vi "Begin.vi"(8 "error in":errorcluster) -> (0 "error out":errorcluster)   [LabVIEW 2019]
doc: "Called before other user functions, this VI is expected to open initial I/O refnums, load in file data, and do all program initialization. Notice that the <B>error out</B> terminal is simply used for data flow. Wiring it to other structures or subVIs ensures that this VI runs first."
uses:
  <vilib>/Rock Robotics/WPI/DriverStation/WPI_DriverStationRobotMode2.ctl
  <vilib>/Rock Robotics/WPI/Joystick/WPI_JoystickDeviceEnum.ctl
  <vilib>/Rock Robotics/SystemInterfaces/DIO/FPGA_DIOPWMChannel.ctl
  <vilib>/Rock Robotics/SystemInterfaces/DIO/FPGA_DIORelayChannel.ctl
  <vilib>/Rock Robotics/WPI/Solenoid/WPI_SolenoidChannel.ctl
  <vilib>/Rock Robotics/SystemInterfaces/DIO/FPGA_DIOChannel.ctl
  <vilib>/Rock Robotics/SystemInterfaces/i2clib/i2c_bus.ctl
  <vilib>/Rock Robotics/SystemInterfaces/AI/FPGA_AIChannel.ctl
  <vilib>/Rock Robotics/SystemInterfaces/spilib/spi_bus.ctl
  Robot Global Data.vi
  <vilib>/Rock Robotics/WPI/MotorControl/WPI_MotorControlOpen SPARK.vi
  <vilib>/Rock Robotics/WPI/MotorControl/WPI_MotorControlOpen VictorSPX.vi
  <vilib>/Rock Robotics/WPI/Solenoid/WPI_SolenoidOpenSingle.vi
  <vilib>/Rock Robotics/WPI/Counter/WPI_CounterDigitalInputToDigitalSource.vi
  Program Files/navX.Library.v2/navX Library v2/IO/Open/Z900_navX_Open_SPI.vi
  Program Files/navX.Library.v2/navX Library v2/navX Library v2.lvlib
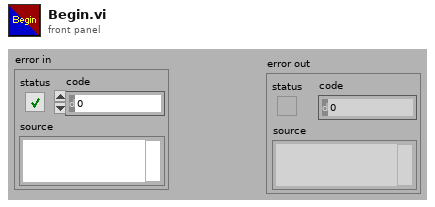
[diagram p1: front panel]
types:
  T1 = typedef "WPI_DriverStationRobotMode2.ctl" = enum16{"Autonomous Disabled", "Autonomous Enabled", "Teleop Disabled", "Teleop Enabled", "Disconnected", "Finish", "Test Disabled", "Test Enabled", "Emergency Stopped"}
  T2 = typedef "WPI_JoystickDeviceEnum.ctl" = enum16{"USB 0", "USB 1", "USB 2", "USB 3", "USB 4", "USB 5"}
  T3 = typedef "FPGA_DIORelayChannel.ctl" = enum8{"Relay 0", "Relay 1", "Relay 2", "Relay 3", "Invalid"}
  T4 = typedef "WPI_SolenoidChannel.ctl" = enum8{"Solenoid 0", "Solenoid 1", "Solenoid 2", "Solenoid 3", "Solenoid 4", "Solenoid 5", "Solenoid 6", "Solenoid 7", "Invalid"}
  T5 = typedef "FPGA_DIOPWMChannel.ctl" = enum8{"PWM 0", "PWM 1", "PWM 2", "PWM 3", "PWM 4", "PWM 5", "PWM 6", "PWM 7", "PWM 8", "PWM 9", "PWM MXP 0", "PWM MXP 1", "PWM MXP 2", "PWM MXP 3", "PWM MXP 4", "PWM MXP 5", "PWM MXP 6", "PWM MXP 7", "PWM MXP 8", "PWM MXP 9", "Invalid"}
  T6 = typedef "FPGA_AIChannel.ctl" = enum8{"AI 0", "AI 1", "AI 2", "AI 3", "AI MXP 0", "AI MXP 1", "AI MXP 2", "AI MXP 3", "Invalid"}
  T7 = typedef "spi_bus.ctl" = enum16{"SPI On-Board, CS0", "SPI On-Board, CS1", "SPI On-Board, CS2", "SPI On-Board, CS3", "SPI MXP", "Invalid"}
  T8 = typedef "i2c_bus.ctl" = enum16{"I2C On-Board", "I2C MXP", "Invalid"}
  T9 = typedef "WPI_JoystickDevRef.ctl" = cluster{"Device":T2}
  T10 = typedef "WPI_MotorControlDeviceRef.ctl" = cluster{"DeviceStatus":errorcluster, "Type":T11, "PWM":cluster{"PWM Channel":T5, "DeadBand":T12}, "CAN":cluster{"Device Number":u8, "SetOutput VI Ref":variant, "GetOutput VI Ref":variant, "Enable VI Ref":variant, "Disable VI Ref":variant, "Data":variant}, "Invert":bool, "DIO PWM":cluster{"PWM \"Enable\" Channel":T5, "DIOChannel":T13, "PWM Rate":dbl}}
  T11 = typedef "WPI_MotorControlType.ctl" = enum16{"PWM", "CAN", "DIO PWM"}
  T12 = typedef "WPI_PWMDeadband.ctl" = cluster{"Name":string, "maxPositivePwm":i32, "minPositivePwm":i32, "centerPwm":i32, "maxNegativePwm":i32, "minNegativePwm":i32, "angularRange":u16}
  T13 = typedef "FPGA_DIOChannel.ctl" = enum8{"DIO 0", "DIO 1", "DIO 2", "DIO 3", "DIO 4", "DIO 5", "DIO 6", "DIO 7", "DIO 8", "DIO 9", "DIO MXP 0", "DIO MXP 1", "DIO MXP 2", "DIO MXP 3", "DIO MXP 4", "DIO MXP 5", "DIO MXP 6", "DIO MXP 7", "DIO MXP 8", "DIO MXP 9", "DIO MXP 10", "DIO MXP 11", "DIO MXP 12", "DIO MXP 13", "DIO MXP 14", "DIO MXP 15", "SPI Port CS1", "SPI Port CS2", "SPI Port CS3", "SPI Port MISO", "SPI Port MOSI", "Invalid"}
  T14 = typedef "WPI_RelayDevRef.ctl" = cluster{"DevStatus":errorcluster, "Relay Channel":T3, "Relay Direction":T15}
  T15 = typedef "WPI_RelayDirection.ctl" = enum16{"Both directions", "Forward only", "Reverse only"}
  T16 = typedef "WPI_CompressorDevRef.ctl" = cluster{"DevStatus":errorcluster, "Pneumatics Control Module":u8}
  T17 = typedef "WPI_SolenoidDevRef.ctl" = cluster{"DevStatus":errorcluster, "Pneumatics Control Module":u8, "Forward Solenoid Channel":T4, "Reverse Solenoid Channel":T4}
  T18 = typedef "WPI_AnalogChannelDevRef.ctl" = cluster{"DevStatus":errorcluster, "Analog Channel":T6}
  T19 = typedef "WPI_DigitalInputDevRef.ctl" = cluster{"DevStatus":errorcluster, "DIO Channel":T13}
  T20 = typedef "Color Sensor V3 DevRef.ctl" = cluster{"I2CDevRef":T21}
  T21 = typedef "WPI_I2CDevRef.ctl" = cluster{"DevStatus":errorcluster, "Device Address":u8, "Handle":i32, "I2C Bus":T8}
  T22 = typedef "FPGA_CounterEncoderSourceConvertionLVSourceType.ctl" = cluster{"DevStatus":errorcluster, "AnalogTriggerMode?":bool, "DigitalMode":cluster{"DIO Channel":T23}, "AnalogTriggerMode":cluster{"AnalogTriggerIndex":T24, "OutputType":T25}}
  T23 = typedef "FPGA_DIODigitalSourceChannel.ctl" = enum8{"DIO 0", "DIO 1", "DIO 2", "DIO 3", "DIO 4", "DIO 5", "DIO 6", "DIO 7", "DIO 8", "DIO 9", "DIO MXP 0", "DIO MXP 1", "DIO MXP 2", "DIO MXP 3", "DIO MXP 4", "DIO MXP 5", "DIO MXP 6", "DIO MXP 7", "DIO MXP 8", "DIO MXP 9", "DIO MXP 10", "DIO MXP 11", "DIO MXP 12", "DIO MXP 13", "DIO MXP 14", "DIO MXP 15", "SPI Port CS1", "SPI Port CS2", "SPI Port CS3", "SPI Port MISO", "SPI Port MOSI", "Disabled"}
  T24 = typedef "FPGA_AnalogTriggerIndex.ctl" = enum8{"Trig 0", "Trig 1", "Trig 2", "Trig 3", "Trig 4", "Trig 5", "Trig 6", "Trig 7", "Invalid"}
  T25 = typedef "FPGA_AnalogTriggerOutType.ctl" = enum16{"InWindow", "TriggerState", "Rising", "Falling"}
  T26 = typedef "WPI_EncoderDevRef.ctl" = cluster{"DevStatus":errorcluster, "EncoderIndex":T27, "CounterIndex":T28, "DistancePerCount":dbl, "Decoding Type":T29}
  T27 = typedef "FPGA_EncoderIdx.ctl" = enum8{"Enc 0", "Enc 1", "Enc 2", "Enc 3", "Enc 4", "Enc 5", "Enc 6", "Enc 7", "Invalid"}
  T28 = typedef "FPGA_CounterCtrSystemIndex.ctl" = enum8{"Ctr 0", "Ctr 1", "Ctr 2", "Ctr 3", "Ctr 4", "Ctr 5", "Ctr 6", "Ctr 7", "Invalid"}
  T29 = typedef "WPI_EncoderType.ctl" = enum16{"1x", "2x", "4x"}
  T30 = typedef "navX Library v2.lvlib/Z900_navX_DeviceTypeDef.ctl" = cluster{"Interface":cluster{"Protocol":T31, "Update Rate (4Hz-100Hz)":u8, "navX Open TypeDef":variant}, "Notify Packet":refnum<notifier>, "Loop VI Refnum":refnum<vi>, "Ready to Close Occurrence Refnum":refnum<k4>}
  T31 = typedef "navX Library v2.lvlib/Z900_navX_ProtocolTypeDef.ctl" = enum16{"SERIAL", "I2C", "SPI"}
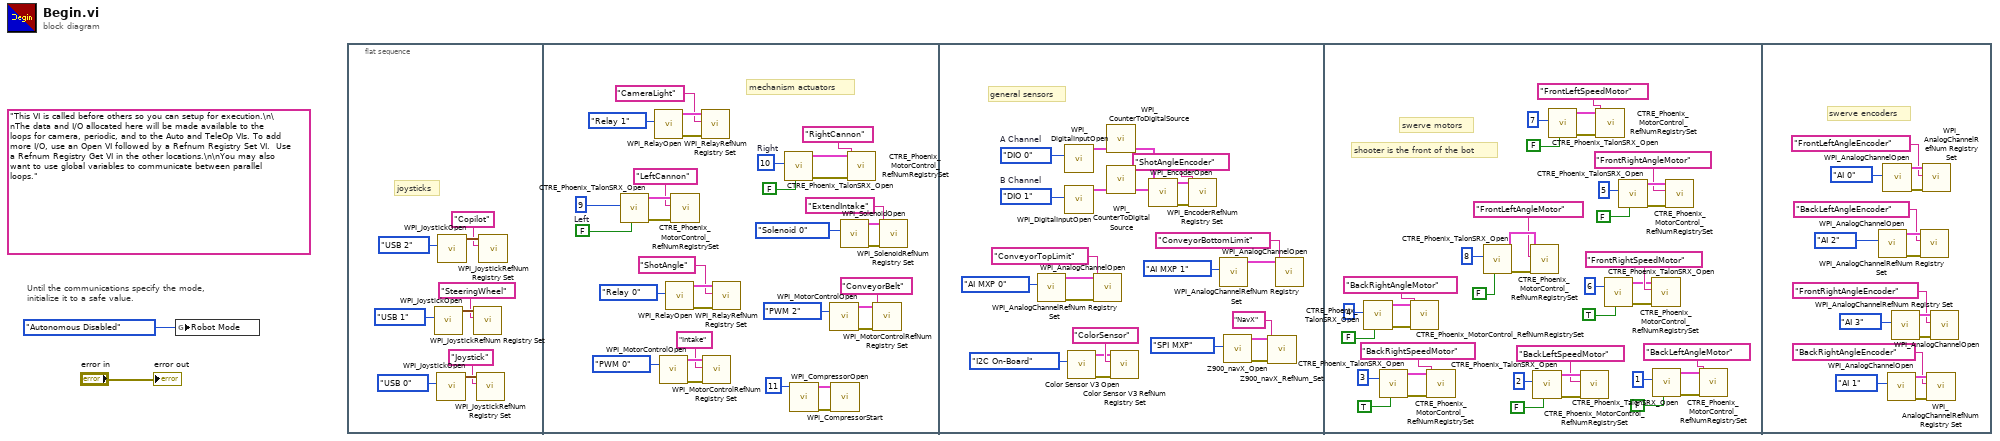
[diagram p0: block diagram]
diagram:
  (unwired) "This VI is called before others so you can setup for execution.\n\nThe data and I/O allocated here will be made available to the loops for camera, periodic, and to the Auto and TeleOp VIs. To add more I/O, use an Open VI followed by a Refnum Registry Set VI.  Use a Refnum Registry Get VI in the other locations.\n\nYou may also want to use global variables to communicate between parallel loops."
  # "Until the communications specify the mode,\ninitialize it to a safe value."
  n1 = global write "Robot Global Data.vi" "Robot Mode"(WPI_DriverStationRobotMode2."Autonomous Disabled" ("Robot Mode")) -> ()
  n2 = flat-sequence {
    frame #0 {
      # "joysticks"
      n3 = call <vilib>:"WPI_JoystickOpen.vi"("JoystickDevice"=WPI_JoystickDeviceEnum."USB 1") -> ("JoystickDevRef"=w7:T9)  [unwired: 10 in]
      n4 = call <vilib>:"WPI_JoystickOpen.vi"("JoystickDevice"=WPI_JoystickDeviceEnum."USB 0") -> ("JoystickDevRef"=w8:T9)  [unwired: 10 in]
      n5 = call <vilib>:"WPI_JoystickOpen.vi"("JoystickDevice"=WPI_JoystickDeviceEnum."USB 2") -> ("JoystickDevRef"=w11:T9)  [unwired: 10 in]
      n6 = call <vilib>:"WPI_JoystickRefNum Registry Set.vi"("refnum name"="SteeringWheel", "JoystickDevRef"=w7) -> ()  [unwired: 8 in, 2 out]
      n7 = call <vilib>:"WPI_JoystickRefNum Registry Set.vi"("refnum name"="Joystick", "JoystickDevRef"=w8) -> ()  [unwired: 8 in, 2 out]
      n8 = call <vilib>:"WPI_JoystickRefNum Registry Set.vi"("refnum name"="Copilot", "JoystickDevRef"=w11) -> ()  [unwired: 8 in, 2 out]
    }
    frame #1 {
      w43 = u8 9  # Left
      w44 = u8 10  # Right
      # "mechanism actuators"
      n9 = call <vilib>:"CTRE_Phoenix_TalonSRX_Open.vi"("Invert"=FALSE, "Device Number"=w43) -> ("error out"=w39:errorcluster, "CAN Talon SRX Ref"=w40:T10)  [unwired: 8 in]
      n10 = call <vilib>:"WPI_RelayOpen.vi"("Relay Channel"=FPGA_DIORelayChannel."Relay 1") -> ("error out"=w18:errorcluster, "RelayDevRef"=w17:T14)  [unwired: 9 in]
      n11 = call-poly <vilib>:"WPI_MotorControlOpen.vi"("PWM Channel"=FPGA_DIOPWMChannel."PWM 0") -> ("error out"=w34:errorcluster, "MotorControlDeviceRef"=w33:T10)  [unwired: 9 in]
      n12 = call <vilib>:"WPI_RelayOpen.vi"("Relay Channel"=FPGA_DIORelayChannel."Relay 0") -> ("error out"=w26:errorcluster, "RelayDevRef"=w25:T14)  [unwired: 9 in]
      n13 = call <vilib>:"CTRE_Phoenix_MotorControl_RefNumRegistrySet.vi"("error in (no error)"=w39, "refnum name"="LeftCannon", "PhoenixMotorControlDevRef"=w40) -> ()  [unwired: 7 in, 2 out]
      n14 = call <vilib>:"WPI_RelayRefNum Registry Set.vi"("error in (no error)"=w18, "refnum name"="CameraLight", "RelayDevRef"=w17) -> ()  [unwired: 7 in, 2 out]
      n15 = call <vilib>:"WPI_MotorControlRefNum Registry Set.vi"("error in (no error)"=w34, "refnum name"="Intake", "MotorControlDevRef"=w33) -> ()  [unwired: 7 in, 2 out]
      n16 = call <vilib>:"WPI_RelayRefNum Registry Set.vi"("error in (no error)"=w26, "refnum name"="ShotAngle", "RelayDevRef"=w25) -> ()  [unwired: 7 in, 2 out]
      n17 = call <vilib>:"CTRE_Phoenix_TalonSRX_Open.vi"("Invert"=FALSE, "Device Number"=w44) -> ("error out"=w36:errorcluster, "CAN Talon SRX Ref"=w37:T10)  [unwired: 8 in]
      n18 = call <vilib>:"WPI_CompressorOpen.vi"("Pneumatics Control Module (0)"=u8 11) -> ("CompressorDevRef"=w13:T16, "error out"=w12:errorcluster)  [unwired: 13 in]
      n19 = call-poly <vilib>:"WPI_MotorControlOpen.vi"("PWM Channel"=FPGA_DIOPWMChannel."PWM 2") -> ("error out"=w30:errorcluster, "MotorControlDeviceRef"=w29:T10)  [unwired: 9 in]
      n20 = call <vilib>:"WPI_CompressorStart.vi"("error in (no error)"=w12, "CompressorDevRef"=w13) -> ()  [unwired: 8 in, 2 out]
      n21 = call-poly <vilib>:"WPI_SolenoidOpen.vi"("Solenoid Channel"=WPI_SolenoidChannel."Solenoid 0") -> ("error out"=w21:errorcluster, "SolenoidDevRef"=w22:T17)  [unwired: 9 in]
      n22 = call <vilib>:"CTRE_Phoenix_MotorControl_RefNumRegistrySet.vi"("error in (no error)"=w36, "refnum name"="RightCannon", "PhoenixMotorControlDevRef"=w37) -> ()  [unwired: 7 in, 2 out]
      n23 = call <vilib>:"WPI_MotorControlRefNum Registry Set.vi"("error in (no error)"=w30, "refnum name"="ConveyorBelt", "MotorControlDevRef"=w29) -> ()  [unwired: 7 in, 2 out]
      n24 = call <vilib>:"WPI_SolenoidRefNum Registry Set.vi"("error in (no error)"=w21, "refnum name"="ExtendIntake", "SolenoidDevRef"=w22) -> ()  [unwired: 7 in, 2 out]
    }
    frame #2 {
      w68 = FPGA_DIOChannel."DIO 1"  # B Channel
      w67 = FPGA_DIOChannel."DIO 0"  # A Channel
      # "general sensors"
      n25 = call <vilib>:"WPI_AnalogChannelOpen.vi"("Analog Channel"=FPGA_AIChannel."AI MXP 0") -> ("error out"=w54:errorcluster, "AIDeviceRef"=w53:T18)  [unwired: 9 in]
      n26 = call <vilib>:"WPI_DigitalInputOpen.vi"("DIO Channel"=w67) -> ("DigitalInputDevRef"=w64:T19)  [unwired: 1 in, 9 out]
      n27 = call <vilib>:"WPI_DigitalInputOpen.vi"("DIO Channel"=w68) -> ("DigitalInputDevRef"=w65:T19)  [unwired: 1 in, 9 out]
      n28 = call <vilib>:"Color Sensor V3 Open.vi"("I2C Bus"=i2c_bus."I2C On-Board") -> ("error out"=w58:errorcluster, "ColorSensorDevRef"=w57:T20)  [unwired: 9 in]
      n29 = call <vilib>:"WPI_AnalogChannelRefNum Registry Set.vi"("error in (no error)"=w54, "refnum name"="ConveyorTopLimit", "AIDeviceRef"=w53) -> ()  [unwired: 7 in, 2 out]
      n30 = call-poly <vilib>:"WPI_CounterToDigitalSource.vi"("DigitalInputDevRef"=w64) -> ("Digital Source"=w63:T22)  [unwired: 6 out]
      n31 = call-poly <vilib>:"WPI_CounterToDigitalSource.vi"("DigitalInputDevRef"=w65) -> ("Digital Source"=w66:T22)  [unwired: 6 out]
      n32 = call <vilib>:"Color Sensor V3 RefNum Registry Set.vi"("error in (no error)"=w58, "refnum name"="ColorSensor", "ColorSensorDevRef"=w57) -> ()  [unwired: 7 in, 2 out]
      n33 = call <vilib>:"WPI_EncoderOpen.vi"("BSource"=w66, "ASource"=w63) -> ("error out"=w62:errorcluster, "EncoderDevRef"=w61:T26)  [unwired: 6 in, 2 out]
      n34 = call <vilib>:"WPI_EncoderRefNum Registry Set.vi"("error in (no error)"=w62, "refnum name"="ShotAngleEncoder", "EncoderDevRef"=w61) -> ()  [unwired: 7 in, 2 out]
      n35 = call <vilib>:"WPI_AnalogChannelOpen.vi"("Analog Channel"=FPGA_AIChannel."AI MXP 1") -> ("AIDeviceRef"=w46:T18)  [unwired: 9 in, 1 out]
      n36 = call-poly "Z900_navX_Open.vi"("SPI Bus"=spi_bus."SPI MXP") -> ("error out"=w48:errorcluster, "navX Device"=w51:T30)  [unwired: 9 in]
      n37 = call "Z900_navX_RefNum_Set.vi"("error in (no error)"=w48, "refnum name"="NavX", "navX Device"=w51) -> ()  [unwired: 7 in, 2 out]
      n38 = call <vilib>:"WPI_AnalogChannelRefNum Registry Set.vi"("refnum name"="ConveyorBottomLimit", "AIDeviceRef"=w46) -> ()  [unwired: 8 in, 2 out]
    }
    frame #3 {
      # "shooter is the front of the bot"
      # "swerve motors"
      n39 = call <vilib>:"CTRE_Phoenix_TalonSRX_Open.vi"("Invert"=FALSE, "Device Number"=u8 4) -> ("error out"=w88:errorcluster, "CAN Talon SRX Ref"=w87:T10)  [unwired: 8 in]
      n40 = call <vilib>:"CTRE_Phoenix_TalonSRX_Open.vi"("Invert"=TRUE, "Device Number"=u8 3) -> ("error out"=w103:errorcluster, "CAN Talon SRX Ref"=w104:T10)  [unwired: 8 in]
      n41 = call <vilib>:"CTRE_Phoenix_MotorControl_RefNumRegistrySet.vi"("error in (no error)"=w88, "refnum name"="BackRightAngleMotor", "PhoenixMotorControlDevRef"=w87) -> ()  [unwired: 7 in, 2 out]
      n42 = call <vilib>:"CTRE_Phoenix_MotorControl_RefNumRegistrySet.vi"("error in (no error)"=w103, "refnum name"="BackRightSpeedMotor", "PhoenixMotorControlDevRef"=w104) -> ()  [unwired: 7 in, 2 out]
      n43 = call <vilib>:"CTRE_Phoenix_TalonSRX_Open.vi"("Invert"=FALSE, "Device Number"=u8 8) -> ("error out"=w76:errorcluster, "CAN Talon SRX Ref"=w75:T10)  [unwired: 8 in]
      n44 = call <vilib>:"CTRE_Phoenix_MotorControl_RefNumRegistrySet.vi"("error in (no error)"=w76, "refnum name"="FrontLeftAngleMotor", "PhoenixMotorControlDevRef"=w75) -> ()  [unwired: 7 in, 2 out]
      n45 = call <vilib>:"CTRE_Phoenix_TalonSRX_Open.vi"("Invert"=FALSE, "Device Number"=u8 2) -> ("error out"=w94:errorcluster, "CAN Talon SRX Ref"=w95:T10)  [unwired: 8 in]
      n46 = call <vilib>:"CTRE_Phoenix_TalonSRX_Open.vi"("Invert"=FALSE, "Device Number"=u8 7) -> ("error out"=w92:errorcluster, "CAN Talon SRX Ref"=w93:T10)  [unwired: 8 in]
      n47 = call <vilib>:"CTRE_Phoenix_MotorControl_RefNumRegistrySet.vi"("error in (no error)"=w94, "refnum name"="BackLeftSpeedMotor", "PhoenixMotorControlDevRef"=w95) -> ()  [unwired: 7 in, 2 out]
      n48 = call <vilib>:"CTRE_Phoenix_MotorControl_RefNumRegistrySet.vi"("error in (no error)"=w92, "refnum name"="FrontLeftSpeedMotor", "PhoenixMotorControlDevRef"=w93) -> ()  [unwired: 7 in, 2 out]
      n49 = call <vilib>:"CTRE_Phoenix_TalonSRX_Open.vi"("Invert"=TRUE, "Device Number"=u8 6) -> ("error out"=w101:errorcluster, "CAN Talon SRX Ref"=w102:T10)  [unwired: 8 in]
      n50 = call <vilib>:"CTRE_Phoenix_TalonSRX_Open.vi"("Invert"=FALSE, "Device Number"=u8 5) -> ("error out"=w86:errorcluster, "CAN Talon SRX Ref"=w85:T10)  [unwired: 8 in]
      n51 = call <vilib>:"CTRE_Phoenix_MotorControl_RefNumRegistrySet.vi"("error in (no error)"=w101, "refnum name"="FrontRightSpeedMotor", "PhoenixMotorControlDevRef"=w102) -> ()  [unwired: 7 in, 2 out]
      n52 = call <vilib>:"CTRE_Phoenix_TalonSRX_Open.vi"("Invert"=FALSE, "Device Number"=u8 1) -> ("error out"=w78:errorcluster, "CAN Talon SRX Ref"=w77:T10)  [unwired: 8 in]
      n53 = call <vilib>:"CTRE_Phoenix_MotorControl_RefNumRegistrySet.vi"("error in (no error)"=w86, "refnum name"="FrontRightAngleMotor", "PhoenixMotorControlDevRef"=w85) -> ()  [unwired: 7 in, 2 out]
      n54 = call <vilib>:"CTRE_Phoenix_MotorControl_RefNumRegistrySet.vi"("error in (no error)"=w78, "refnum name"="BackLeftAngleMotor", "PhoenixMotorControlDevRef"=w77) -> ()  [unwired: 7 in, 2 out]
    }
    frame #4 {
      # "swerve encoders"
      n55 = call <vilib>:"WPI_AnalogChannelOpen.vi"("Analog Channel"=FPGA_AIChannel."AI 2") -> ("error out"=w119:errorcluster, "AIDeviceRef"=w120:T18)  [unwired: 9 in]
      n56 = call <vilib>:"WPI_AnalogChannelOpen.vi"("Analog Channel"=FPGA_AIChannel."AI 0") -> ("error out"=w123:errorcluster, "AIDeviceRef"=w124:T18)  [unwired: 9 in]
      n57 = call <vilib>:"WPI_AnalogChannelOpen.vi"("Analog Channel"=FPGA_AIChannel."AI 1") -> ("error out"=w111:errorcluster, "AIDeviceRef"=w112:T18)  [unwired: 9 in]
      n58 = call <vilib>:"WPI_AnalogChannelOpen.vi"("Analog Channel"=FPGA_AIChannel."AI 3") -> ("error out"=w115:errorcluster, "AIDeviceRef"=w116:T18)  [unwired: 9 in]
      n59 = call <vilib>:"WPI_AnalogChannelRefNum Registry Set.vi"("error in (no error)"=w119, "refnum name"="BackLeftAngleEncoder", "AIDeviceRef"=w120) -> ()  [unwired: 7 in, 2 out]
      n60 = call <vilib>:"WPI_AnalogChannelRefNum Registry Set.vi"("error in (no error)"=w123, "refnum name"="FrontLeftAngleEncoder", "AIDeviceRef"=w124) -> ()  [unwired: 7 in, 2 out]
      n61 = call <vilib>:"WPI_AnalogChannelRefNum Registry Set.vi"("error in (no error)"=w111, "refnum name"="BackRightAngleEncoder", "AIDeviceRef"=w112) -> ()  [unwired: 7 in, 2 out]
      n62 = call <vilib>:"WPI_AnalogChannelRefNum Registry Set.vi"("error in (no error)"=w115, "refnum name"="FrontRightAngleEncoder", "AIDeviceRef"=w116) -> ()  [unwired: 7 in, 2 out]
    }
  }
  "error out" <- "error in"
